vi "Storage Data.vi"(8 "error in (no error)":errorcluster, 10 "Data In":u16[][](array[numeric]), 11 "2D U16 DVR Array in":refnum<class "2D U16 DVR Array.lvclass">) -> (0 "error out":errorcluster, 3 "2D U16 DVR Array out":refnum<class "2D U16 DVR Array.lvclass">)   [LabVIEW 2019, in "2D U16 DVR Array.lvclass"]
uses:
  2D U16 DVR Array.lvclass
  2D U16 DVR Array.lvclass/2D U16 DVR Array.ctl
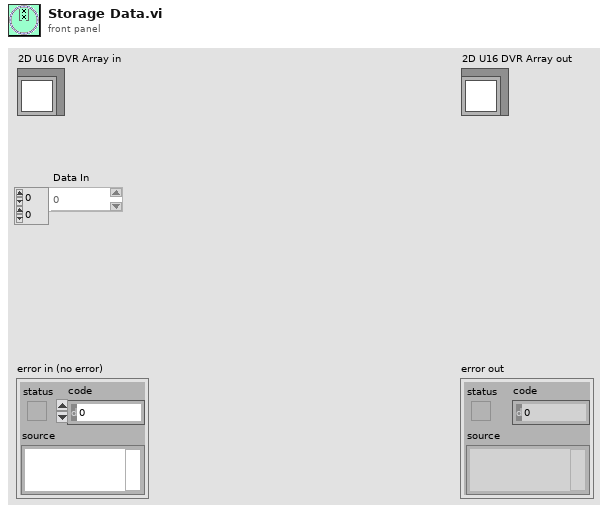
[diagram p1: front panel]
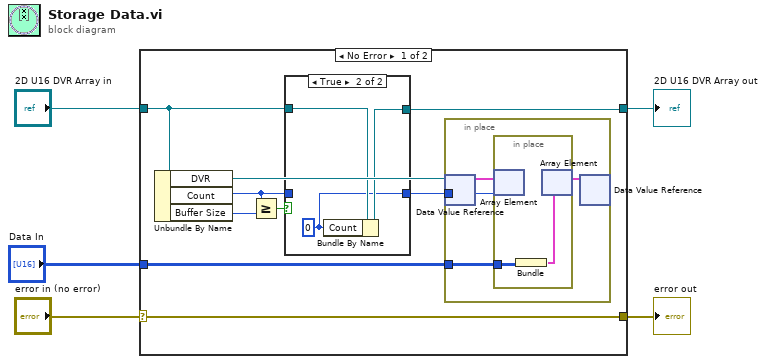
[diagram p0: block diagram]
diagram:
  n1 = case shown="No Error" "error in (no error)" {
    selector: "error in (no error)" -> [w14 w27]
    tunnel: [w14 w27] -> w4
    tunnel: [w9 w26] -> w2
    tunnel: "2D U16 DVR Array in" -> [w11 w26]
    tunnel: "Data In" -> [w6 _]
    frame No Error {
      n2 = Unbundle By Name(w11) -> ("DVR"=w8:refnum<data-value>, "Count"=w10:i32, "Buffer Size"=w13:i32)
      n3 = Greater Or Equal?(x=w10, y=w13) -> (x >= y?=w12:bool)
      n4 = case shown="True" w12 {
        tunnel: w11 -> [w22 w25]
        tunnel: [w22 w24] -> w9
        tunnel: w10 -> [w21 _]
        tunnel: [w21 w23] -> w7
        frame False {
        }
        frame True {
          w23 = 0 ("Count")
          n5 = Bundle By Name(cluster=w25, "Count"=w23) -> (w24:refnum<class "2D U16 DVR Array.lvclass">)
        }
      }
      n6 = in-place {
        in-place-border: w7 -> [w17]
        in-place-border: w6 -> [w16]
        n7 = in-place-dvr #1(w8) -> (w18:cluster{u16[][]}[])  [unwired: 1 out]
        n8 = in-place {
          in-place-border: w16 -> [w20]
          n9 = in-place-array #2(w18, w17) -> ()  [unwired: 1 out]
          n10 = Bundle("Data In"=w20) -> (w19:cluster{"Data In":u16[][]})  [unwired: 1 in]
          n11 = in-place-array #2(w19) -> (w15:cluster{u16[][]}[])  [unwired: 1 out]
        }
        n12 = in-place-dvr #1(w15) -> ()  [unwired: 2 out]
      }
    }
    frame Error {
    }
  }
  "error out" <- w4
  "2D U16 DVR Array out" <- w2
